vi "ziExample-Module-SWtrigger.vi"() -> ()   [LabVIEW 2009]
doc: "Control a Zurich instrument device via the LabOne Labview API. \nRequirements: Zurich Instruments MFLI, HF2 or UHFLI \nThis example shows how to start a software trigger module and retrieve the Data.\n\n© Zurich Instruments AG, www.zhinst.com"
uses:
  <instrlib>/Zurich Instruments LabOne/Public/Modules/ziModSetValueBinary.vi
  <instrlib>/Zurich Instruments LabOne/Public/Configure/ziSetValueDoubleArray.vi
  <instrlib>/Zurich Instruments LabOne/Public/Modules/ziModSetValueDouble.vi
  <instrlib>/Zurich Instruments LabOne/Public/Modules/ziModGetAuxinData.vi
  <instrlib>/Zurich Instruments LabOne/Public/Modules/ziModGetCounterData.vi
  <instrlib>/Zurich Instruments LabOne/Public/Modules/ziModGetDemodData.vi
  <instrlib>/Zurich Instruments LabOne/Public/Utility/ziTicksToS_vector.vi
  <instrlib>/Zurich Instruments LabOne/Public/Utility/ziTicksToS_single.vi
  <instrlib>/Zurich Instruments LabOne/Public/Modules/ziModGetImpedanceData.vi
  <instrlib>/Zurich Instruments LabOne/Zurich Instruments LabOne.lvlib
panel:
  out "Slide":dbl(slide) scale=0.0..1.0
  in  "subscribe":string="demods/0/sample"
  out "Grid DEMOD X":dbl[][](graph)
  out "Error Out":errorcluster
  in  "stop":bool
  in  "run":bool caption="Run"
  in  "TriggerModulSetup":T1={"holdoff/time"=0.2, "holdoff/count"=0.0, "delay"=-0.00125, "duration"=0.01, "pulse/min"=0.0, "pulse/max"=0.0, "type"=1, "edge"=1, "count"=5.0, "bits"=1.0, "bitmask"=1.0, "triggernode"="demods/0/sample.R", "bandwidth"=0.0, "hysteresis"=0.003, "level"=0.03, "grid/mode"=0.0, "grid/operation"=0.0, "grid/cols"=100, "grid/rows"=100, "grid/direction"=0.0, "grid/repetitions"=1.0} {"grid/direction" items=["Forward", "Reverse", "Bi-directional"]; "grid/operation" items=["Replace", "Average"]; "grid/mode" items=["OFF", "Nearest", "Linear"]; "level" format="%#_6p"; "hysteresis" format="%#_6p"; "bandwidth" format="%#_6p"; "edge" items=["positive"=1, "negative"=2, "both"=3]; "type" items=["edge"=1, "digital"=2, "pulse"=3, "tracking edge"=4, "HW Trigger"=6, "tracking pulse"=7]}
  out "Demod X":T2(graph)
  in  "Address":string="DEV"
  out "Selected Device":string
  # "ziExample-SweepModul.vi\nRequirements: \n- HF2LI, UHFLI or MFLI \n- MD Option\nsee block diagram for VI description"
  # "Tested Instruments:\n- HF2LI\n- UHFLI\n- MFLI"
  # "Trigger Settings"
  # "edge/pulse/tracking edge/tracking pulse"
  # "only for tracking mode"
  # "digital"
  # "Horizontal"
  # "only for pulse/tracking pulse"
  # "only for pulse/tracking pulse"
  # "Grid Mode"
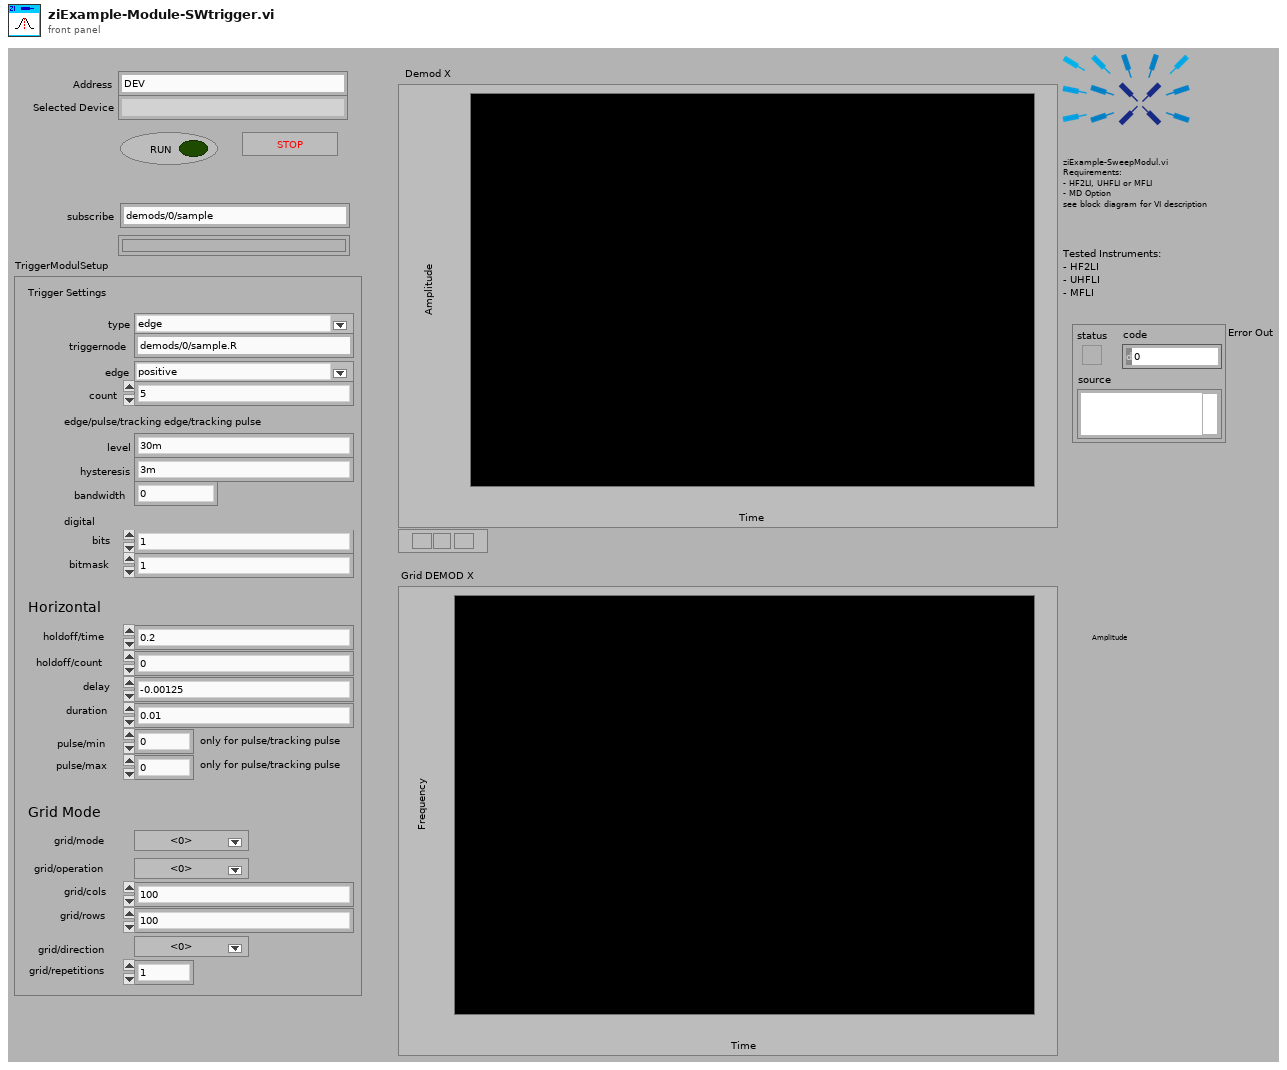
[diagram p1: front panel]
types:
  T1 = cluster{"holdoff/time":dbl, "holdoff/count":dbl, "delay":dbl, "duration":dbl, "pulse/min":dbl, "pulse/max":dbl, "type":u16, "edge":u16, "count":dbl, "bits":dbl, "bitmask":dbl, "triggernode":string, "bandwidth":dbl, "hysteresis":dbl, "level":dbl, "grid/mode":dbl, "grid/operation":dbl, "grid/cols":u32, "grid/rows":u32, "grid/direction":dbl, "grid/repetitions":dbl}
  T2 = cluster{"Timestamp(s)":dbl[], "X (Vrms)":dbl[]}[]
  T3 = typedef "Zurich Instruments LabOne.lvlib/ziTypeHandle.ctl" = cluster{"handleValid":bool, "Conn":u64, "Path Prefix":string, "Handle":u64, "Connected":bool, "Clockbase(s)":dbl}
  T4 = typedef "Zurich Instruments LabOne.lvlib/ziTypeModHandle.ctl" = cluster{"handleValid":bool, "Conn":u64, "ModHandle":u64, "moduleID":string, "Path Prefix":string}
  T5 = typedef "Zurich Instruments LabOne.lvlib/ziTypeModResults.ctl" = cluster{"PathArray":string[], "ValueType":T6, "NoOfResults":u64, "HeaderType":enum16{"HEADER_TYPE_NONE", "HEADER_TYPE_SWTRIGGER", "HEADER_TYPE_SWEEPER"}, "ziSWTriggerHeader":T7[], "ziSweeperHeader":T8[]}
  T6 = typedef "Zurich Instruments LabOne.lvlib/ziTypePollType.ctl" = enum16{"NONE", "DOUBLE_DATA", "INTEGER_DATA", "DEMOD_SAMPLE", "SCOPE_WAVE_HF2", "AUXIN_SAMPLE", "DIO_SAMPLE", "BYTE_ARRAY", "PWA_WAVE", "9", "10", "11", "12", "13", "14", "15", "TREE_CHANGE_DEPRI", "17", "ERROR", "19", "20", "21", "22", "23", "24", "25", "26", "27", "28", "29", "30", "31", "DOUBLE_DATA_TS", "INTEGER_DATA_TS", "34", "SCOPE_WAVE", "36", "37", "BYTE_ARRAY_TS", "39", "40", "41", "42", "43", "44", "45", "CNT_DATA", "47", "TREE_CHANGE", "49", "50", "51", "52", "53", "54", "55", "56", "57", "58", "59", "60", "61", "62", "63", "SWEEPER_DATA", "SPECTRUM_DATA", "ADVISOR_DATA", "67", "IMP_DATA"}
  T7 = typedef "Zurich Instruments LabOne.lvlib/ziTypeModSWTriggerHeader.ctl" = cluster{"HeaderType":enum8{"HEADER_TYPE_NONE", "HEADER_TYPE_SWTRIGGER", "HEADER_TYPE_SWEEPER"}, "triggerStart":u64, "triggerNumber":u64, "cols":u32, "rows":u32}
  T8 = typedef "Zurich Instruments LabOne.lvlib/ziTypeModSweeperHeader.ctl" = cluster{"HeaderType":enum8{"HEADER_TYPE_NONE", "HEADER_TYPE_SWTRIGGER", "HEADER_TYPE_SWEEPER"}, "sampleFormat":u8}
  T9 = typedef "ziTypeDemodSampleExGrid.ctl" = cluster{"Timestamps (ticks)":u64[][], "X (Vrms)":dbl[][], "Y (Vrms)":dbl[][], "Osc Phase (rad)":dbl[][], "Freq (Hz)":dbl[][], "DIO":u32[][], "Aux In 0 (V)":dbl[][], "Aux In 1 (V)":dbl[][], "Trigger":u32[][]}
  T10 = typedef "ziTypeDemodSampleEx.ctl" = cluster{"Timestamps (ticks)":u64[], "X (Vrms)":dbl[], "Y (Vrms)":dbl[], "Osc Phase (rad)":dbl[], "Freq (Hz)":dbl[], "DIO":u32[], "Aux In 0 (V)":dbl[], "Aux In 1 (V)":dbl[], "Trigger":u32[]}
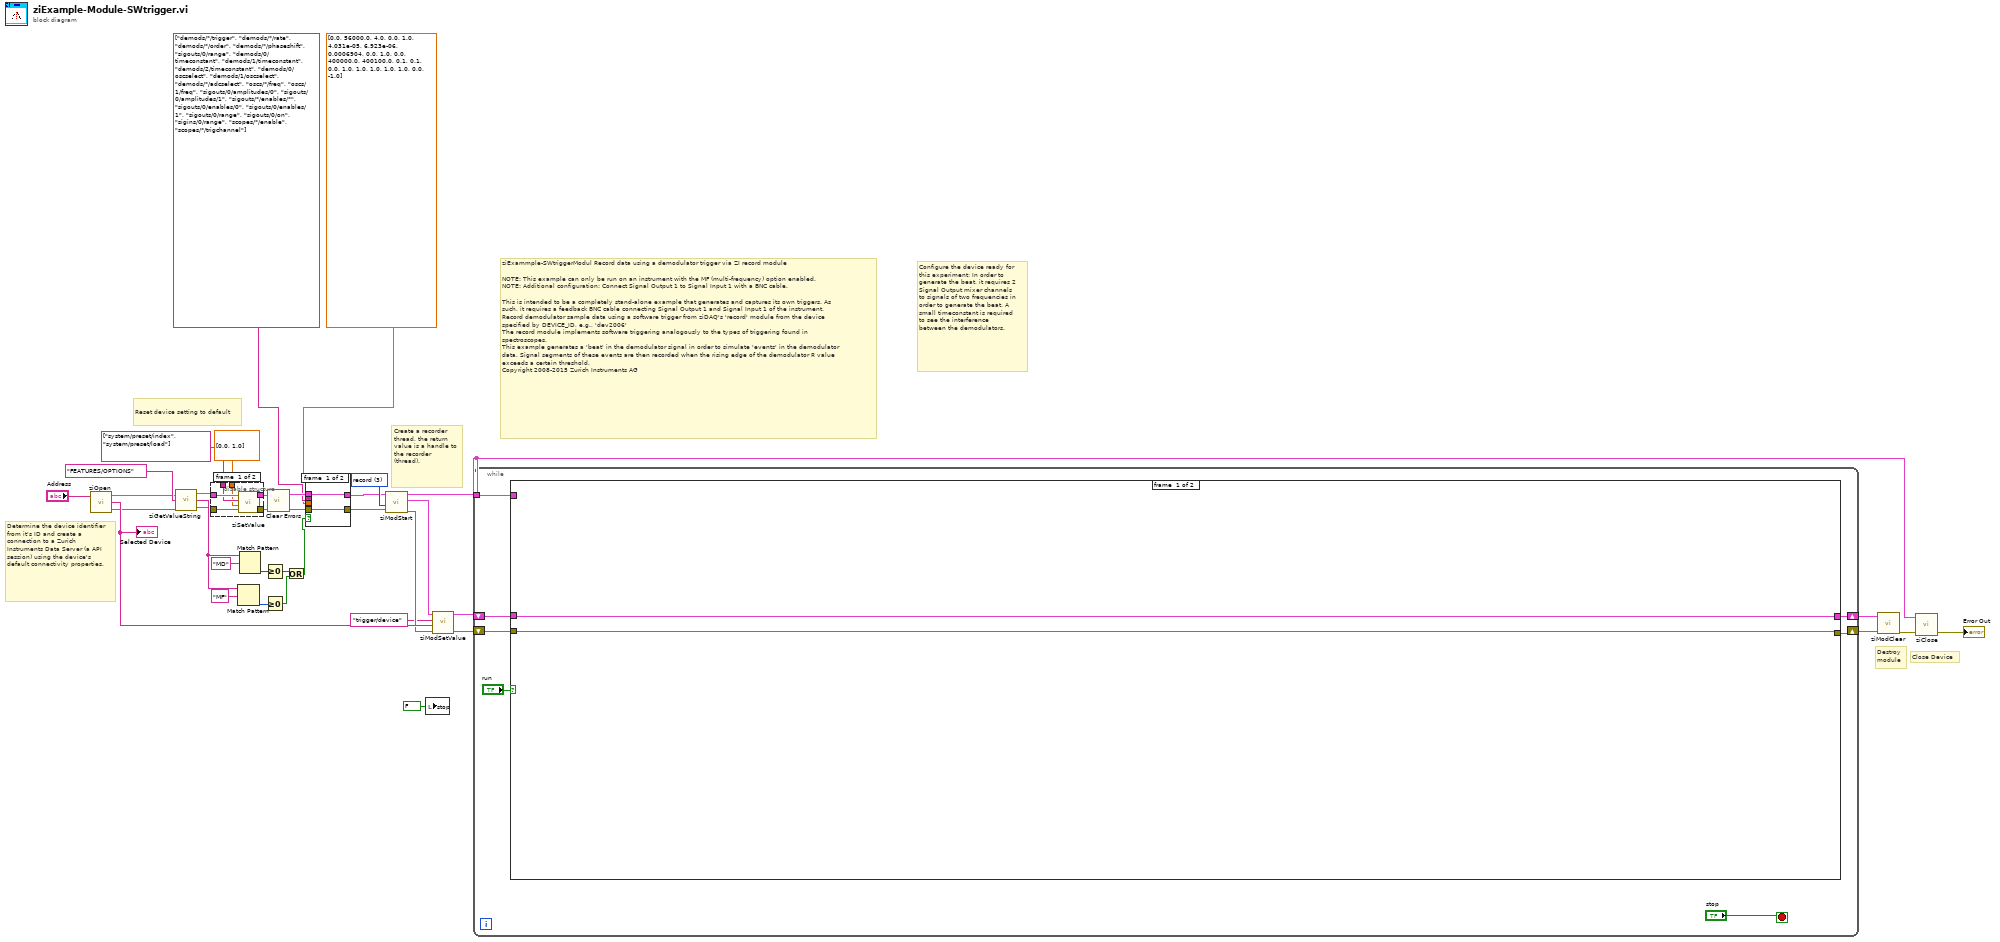
[diagram p0: block diagram]
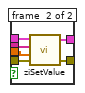
[diagram p2: hidden frame]
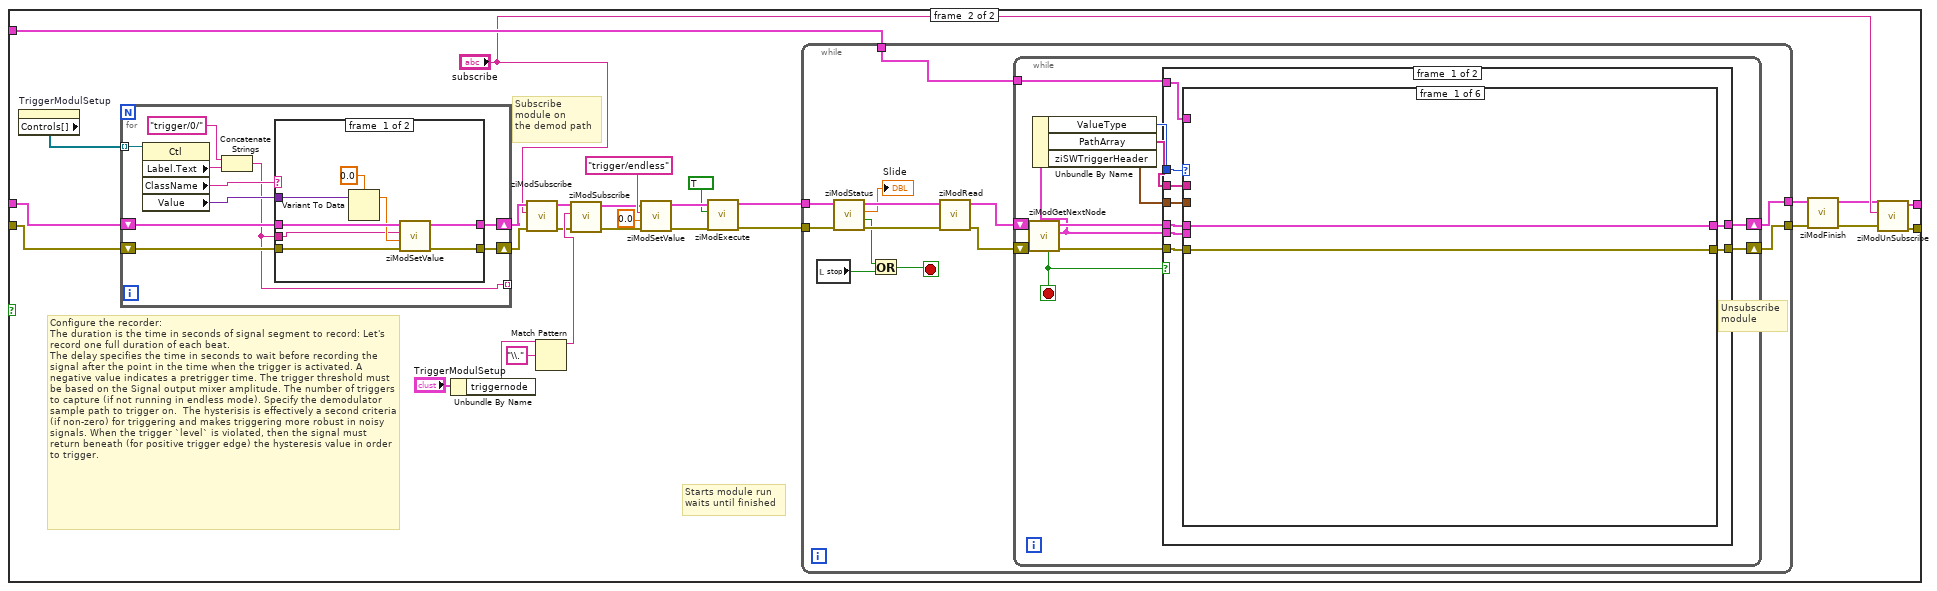
[diagram p4: hidden frame]
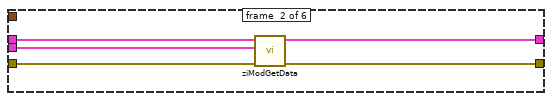
[diagram p5: hidden frame]
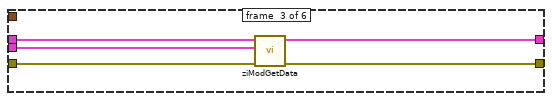
[diagram p6: hidden frame]
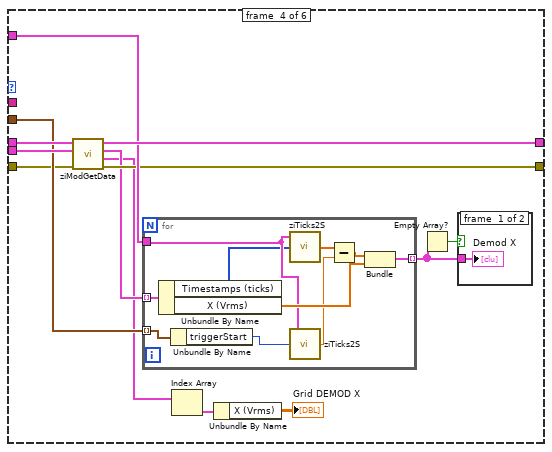
[diagram p7: hidden frame]
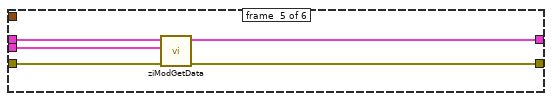
[diagram p9: hidden frame]
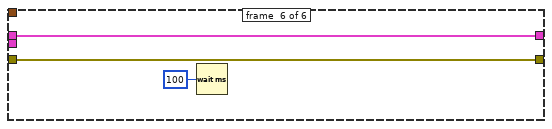
[diagram p10: hidden frame]
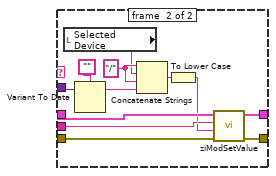
[diagram p12: hidden frame]
diagram:
  w34 = u16 3 items=["sweep", "zoomFFT", "deviceSettings", "record", "pllAdvisor", "pidAdvisor"] ("moduleID")
  # "ziExammple-SWtriggerModul Record data using a demodulator trigger via ZI record module\n\nNOTE: This example can only be run on an instrument with the MF (multi-frequency) option enabled. \nNOTE: Additional configuration: Connect Signal Output 1 to Signal Input 1 with a BNC cable.\n\nThis is intended to be a completely stand-alone example that generates and captures its own triggers. As such, it requires a feedback BNC cable connecting Signal Output 1 and Signal Input 1 of the instrument.\nRecord demodulator sample data using a software trigger from ziDAQ's 'record' module from the device specified by DEVICE_ID, e.g., 'dev2006' \nThe record module implements software triggering analogously to the types of triggering found in spectroscopes.\nThis example generates a 'beat' in the demodulator signal in order to simulate 'events' in the demodulator data. Signal segments of these events are then recorded when the rising edge of the demodulator R value exceeds a certain threshold.\nCopyright 2008-2015 Zurich Instruments AG"
  # "Configure the device ready for this experiment: In order to generate the beat, it requires 2 Signal Output mixer channels to signals of two frequencies in order to generate the beat. A small timeconstant is required to see the interference between the demodulators."
  # "Reset device setting to default"
  # "Destroy\nmodule"
  # "Create a recorder thread, the return value is a handle to the recorder (thread)."
  # "Close Device"
  # "Determine the device identifier from it's ID and create a connection to a Zurich Instruments Data Server (a API session) using the device's default connectivity properties."
  n1 = call <instrlib>:"ziOpen.vi"("Address"="Address") -> ("Error Out"=w5:errorcluster, "Selected Device"=w35:string, "HandleOut"=w4:T3)  [unwired: 1 in, 2 out]
  "Selected Device" <- w35
  n2 = call <instrlib>:"ziGetValueString.vi"("error in"=w5, "Path"="FEATURES/OPTIONS", "Handle In"=w4) -> ("error out"=w2:errorcluster, "Value"=w10:string, "Handle Out"=w3:T3)
  n3 = disable-structure shown="Enabled" {
    disable-tunnel: w3 -> [w42 w44]
    disable-tunnel: [w41 w44] -> w27
    disable-tunnel: [w40 w43] -> w26
    disable-tunnel: w2 -> [w39 w43]
    disable-tunnel: string[] ["system/preset/index", "system/preset/load"] -> [w38 _]
    disable-tunnel: dbl[] [0.0, 1.0] -> [w37 _]
    frame #0 {
      n4 = call-poly <instrlib>:"ziSetValue.vi"("Error In"=w39, "Values"=w37, "Paths"=w38, "Handle In"=w42) -> ("Error Out"=w40:errorcluster, "Handle Out"=w41:T3)  [unwired: 1 in]
    }
    frame #1 {
    }
  }
  n5 = Match Pattern(string=w10, regular expression="MF") -> (offset past match=w8:i32)  [unwired: 1 in, 3 out]
  n6 = Match Pattern(string=w10, regular expression="MD") -> (offset past match=w11:i32)  [unwired: 1 in, 3 out]
  n7 = Greater Or Equal To 0?(x=w11) -> (x >= 0?=w7:bool)
  n8 = Greater Or Equal To 0?(x=w8) -> (x >= 0?=w6:bool)
  n9 = call <vilib>:"Clear Errors.vi"("error in (no error)"=w26) -> ("error out"=w16:errorcluster)  [unwired: 6 in]
  n10 = Or(x=w7, y=w6) -> (x .or. y?=w1:bool)
  n11 = case shown="True" w1 {
    tunnel: [w46 w52] -> w30
    tunnel: [w45 w51] -> w29
    tunnel: w27 -> [w46 w50]
    tunnel: string[] ["demods/*/trigger", "demods/*/rate", "demods/*/order", "demods/*/phaseshift", "sigouts/0/range", "demods/0/timeconstant", "demods/1/timeconstant", "demods/2/timeconstant", "demods/0/oscselect", "demods/1/oscselect", "demods/*/adcselect", "oscs/*/freq", "oscs/1/freq", "sigouts/0/amplitudes/0", "sigouts/0/amplitudes/1", "sigouts/*/enables/*", "sigouts/0/enables/0", "sigouts/0/enables/1", "sigouts/0/range", "sigouts/0/on", "sigins/0/range", "scopes/*/enable", "scopes/*/trigchannel"] -> [_ w49]
    tunnel: dbl[] [0.0, 56000.0, 4.0, 0.0, 1.0, 4.031e-05, 6.923e-06, 0.0006904, 0.0, 1.0, 0.0, 400000.0, 400100.0, 0.1, 0.1, 0.0, 1.0, 1.0, 1.0, 1.0, 1.0, 0.0, -1.0] -> [_ w48]
    tunnel: w16 -> [w45 w47]
    frame #0 {
    }
    frame #1 {
      n12 = call-poly <instrlib>:"ziSetValue.vi"("Error In"=w47, "Values"=w48, "Paths"=w49, "Handle In"=w50) -> ("Error Out"=w51:errorcluster, "Handle Out"=w52:T3)  [unwired: 1 in]
    }
  }
  n13 = call <instrlib>:"ziModStart.vi"("Error In"=w29, "module Id"=w34, "Handle In"=w30) -> ("Error Out"=w32:errorcluster, "ModHandle Out"=w33:T4, "Handle Out"=w24:T3)  [unwired: 6 in]
  n14 = local write "stop"(FALSE ("stop")) -> ()
  n15 = call-poly <instrlib>:"ziModSetValue.vi"("Error In"=w32, "Data"=w35, "Path"="trigger/device", "ModHandle In"=w33) -> ("Error Out"=w25:errorcluster, "ModHandle Out"=w15:T4)  [unwired: 6 in]
  n16 = while {
    tunnel: w24 -> [w59]
    shift-right: [w54] -> w22
    shift-left: w15 -> [w58]
    shift-right: [w53] -> w23
    shift-left: w25 -> [w57]
    stop <- "stop" stop-if-true
    n17 = case shown="True" "run" {
      tunnel: [w60 w78] -> w54
      tunnel: [w61 w79] -> w53
      tunnel: w59 -> [_ w87]
      tunnel: w58 -> [w60 w83]
      tunnel: w57 -> [w61 w82]
      frame #0 {
      }
      frame #1 {
        # "Starts module run\nwaits until finished"
        # "Configure the recorder:\nThe duration is the time in seconds of signal segment to record: Let's record one full duration of each beat.\nThe delay specifies the time in seconds to wait before recording the signal after the point in the time when the trigger is activated. A negative value indicates a pretrigger time. The trigger threshold must be based on the Signal output mixer amplitude. The number of triggers to capture (if not running in endless mode). Specify the demodulator sample path to trigger on.  The hysterisis is effectively a second criteria (if non-zero) for triggering and makes triggering more robust in noisy signals. When the trigger `level` is violated, then the signal must return beneath (for positive trigger edge) the hysteresis value in order to trigger."
        # "Subscribe\nmodule on\nthe demod path"
        n18 = property on="TriggerModulSetup" class="Clust (strict)"() -> ("Controls[]"=w86:refnum<vi>[])  [unwired: 2 in, 2 out]
        n19 = for {
          tunnel: w86 -> [w179] mode=indexing
          shift-right: [w173] -> w84
          shift-left: w82 -> [w171]
          shift-right: [w174] -> w85
          shift-left: w83 -> [w172]
          tunnel: [w170] -> _ mode=indexing
          n20 = property class="Ctl"(reference=w179) -> ("Label.Text"=w177:string, "ClassName"=w176:string, "Value"=w175:variant)  [unwired: 1 in, 2 out]
          n21 = Concatenate Strings("trigger/0/" ("string"), w177) -> (w170:string)
          n22 = case shown="\"String\"" w176 {
            tunnel: w170 -> [w180 w193]
            tunnel: w175 -> [w187 w198]
            tunnel: [w184 w197] -> w174
            tunnel: [w183 w196] -> w173
            tunnel: w172 -> [w185 w195]
            tunnel: w171 -> [w182 w194]
            frame #0 {
              n23 = Variant To Data(Variant=w187, type=0.0) -> (data=w181:dbl)  [unwired: 1 in, 1 out]
              n24 = call-poly <instrlib>:"ziModSetValue.vi"("Error In"=w182, "Value"=w181, "Path"=w180, "ModHandle In"=w185) -> ("Error Out"=w183:errorcluster, "ModHandle Out"=w184:T4)  [unwired: 6 in]
            }
            frame #1 {
              w192 = "/"
              n25 = local read "Selected Device"() -> (w191:string)
              n26 = Variant To Data(Variant=w198, type="") -> (data=w190:string)  [unwired: 1 in, 1 out]
              n27 = Concatenate Strings(w192, w191, w192, w190) -> (w189:string)
              n28 = To Lower Case(string=w189) -> (all lower case string=w188:string)
              n29 = call-poly <instrlib>:"ziModSetValue.vi"("Error In"=w194, "Data"=w188, "Path"=w193, "ModHandle In"=w195) -> ("Error Out"=w196:errorcluster, "ModHandle Out"=w197:T4)  [unwired: 6 in]
            }
          }
        }
        n30 = Unbundle By Name("TriggerModulSetup") -> ("triggernode"=w72:string)
        n31 = call <instrlib>:"ziModSubscribe.vi"("Error In"=w84, "Path"="subscribe", "ModHandle In"=w85) -> ("Error Out"=w68:errorcluster, "ModHandle Out"=w69:T4)  [unwired: 6 in]
        n32 = Match Pattern(string=w72, regular expression="\\.") -> (before substring=w70:string)  [unwired: 1 in, 3 out]
        n33 = call <instrlib>:"ziModSubscribe.vi"("Error In"=w68, "Path"=w70, "ModHandle In"=w69) -> ("Error Out"=w66:errorcluster, "ModHandle Out"=w67:T4)  [unwired: 6 in]
        n34 = call-poly <instrlib>:"ziModSetValue.vi"("Error In"=w66, "Value"=0.0, "Path"="trigger/endless", "ModHandle In"=w67) -> ("Error Out"=w80:errorcluster, "ModHandle Out"=w81:T4)  [unwired: 6 in]
        n35 = call <instrlib>:"ziModExecute.vi"("Error In"=w80, "Modal (F)"=TRUE, "ziModHandle In"=w81) -> ("Error Out"=w74:errorcluster, "ziModHandle Out"=w75:T4)  [unwired: 5 in, 1 out]
        n36 = while {
          tunnel: w87 -> [w102]
          tunnel: w75 -> [w97]
          tunnel: w74 -> [w96]
          tunnel: [w95] -> w64
          tunnel: [w94] -> w63
          stop <- w90 stop-if-true
          # "Unsubscribe\nmodule"
          n37 = local read "stop"() -> (w92:bool)
          n38 = call <instrlib>:"ziModStatus.vi"("Error In"=w96, "ModHandle IN"=w97) -> ("Error Out"=w98:errorcluster, "Finished?"=w91:bool, "Progress (unity)"=→"Slide":dbl, "ModHandle Out"=w99:T4)  [unwired: 5 in]
          n39 = Or(x=w91, y=w92) -> (x .or. y?=w90:bool)
          n40 = call <instrlib>:"ziModRead.vi"("error in"=w98, "ziModHandle In"=w99) -> ("error out"=w101:errorcluster, "ziModHandle Out"=w100:T4)  [unwired: 8 in]
          n41 = while {
            shift-right: [w109] -> w94
            shift-left: w100 -> [w113]
            shift-right: [w110] -> w95
            shift-left: w101 -> [w114]
            tunnel: w102 -> [w108]
            stop <- w106 stop-if-true
            # "Retrieve results"
            n42 = call <instrlib>:"ziModGetNextNode.vi"("Error In"=w114, "ModHandle In"=w113) -> ("Error Out"=w111:errorcluster, "ModResults"=w104:T5, "ModHandle Out"=w112:T4, "NoData"=w106:bool)  [unwired: 6 in]
            n43 = Unbundle By Name(w104) -> ("ValueType"=w105:T6, "PathArray"=w107:string[], "ziSWTriggerHeader"=w103:T7[])
            n44 = case shown="False" w106 {
              tunnel: w104 -> [w123 _]
              tunnel: w112 -> [w122 w169]
              tunnel: w111 -> [w121 w168]
              tunnel: [w120 w168] -> w110
              tunnel: [w119 w169] -> w109
              tunnel: w105 -> [w118 _]
              tunnel: w108 -> [w117 _]
              tunnel: w107 -> [w116 _]
              tunnel: w103 -> [w115 _]
              frame #0 {
                n45 = case shown="\"DEMOD_SAMPLE\"" w118 {
                  tunnel: w122 -> [w125 w130 w135 w145 w162 w167]
                  tunnel: w123 -> [_ w128 w133 w146 w163 _]
                  tunnel: w121 -> [w124 w129 w134 w141 w160 w166]
                  tunnel: [w124 w126 w131 w144 w161 w166] -> w120
                  tunnel: [w125 w127 w132 w148 w164 w167] -> w119
                  tunnel: w117 -> [_ _ _ w147 _ _]
                  tunnel: w116 -> [_ _ _ _ _ _]
                  tunnel: w115 -> [_ _ _ w142 _ _]
                  frame #0 {
                  }
                  frame #1 {
                    n46 = call-poly <instrlib>:"ziModGetData.vi"("Error In"=w129, "ModResults"=w128, "ModHandle In"=w130) -> ("Error Out"=w126:errorcluster, "ModHandle Out"=w127:T4)  [unwired: 5 in, 2 out]
                  }
                  frame #2 {
                    n47 = call-poly <instrlib>:"ziModGetData.vi"("Error In"=w134, "ModResults"=w133, "ModHandle In"=w135) -> ("Error Out"=w131:errorcluster, "ModHandle Out"=w132:T4)  [unwired: 6 in, 1 out]
                  }
                  frame #3 {
                    n48 = call-poly <instrlib>:"ziModGetData.vi"("Error In"=w141, "ModResults"=w146, "ModHandle In"=w145) -> ("Error Out"=w144:errorcluster, "ModDemodDataGrid"=w140:T9[], "ModDemodData"=w143:T10[], "ModHandle Out"=w148:T4)  [unwired: 5 in]
                    n49 = for {
                      tunnel: w143 -> [w159] mode=indexing
                      tunnel: [w157] -> w137 mode=indexing
                      tunnel: w147 -> [w154]
                      tunnel: w142 -> [w156] mode=indexing
                      n50 = Unbundle By Name(w159) -> ("Timestamps (ticks)"=w152:u64[], "X (Vrms)"=w158:dbl[])
                      n51 = Unbundle By Name(w156) -> ("triggerStart"=w155:u64)
                      n52 = call-poly <instrlib>:"ziTicks2S.vi"("Timestamp (ticks)"=w152, "Handle In"=w154) -> ("Timestamp(s)"=w151:dbl[])  [unwired: 1 in, 2 out]
                      n53 = call-poly <instrlib>:"ziTicks2S.vi"("Timestamp(ticks)"=w155, "Handle In"=w154) -> ("Timestamp(s)"=w153:dbl)  [unwired: 1 in, 2 out]
                      n54 = Subtract(x=w151, y=w153) -> (x-y=w150:dbl[])
                      n55 = Bundle(w150, "X (Vrms)"=w158) -> (w157:cluster{dbl[], "X (Vrms)":dbl[]})  [unwired: 1 in]
                    }
                    n56 = Index Array(array=w140) -> (element=w139:T9)  [unwired: 1 in]
                    n57 = Unbundle By Name(w139) -> ("X (Vrms)"=→"Grid DEMOD X":dbl[][])
                    n58 = Empty Array?(array=w137) -> (empty?=w136:bool)
                    n59 = case shown="False" w136 {
                      tunnel: w137 -> [w149 _]
                      frame #0 {
                        "Demod X" <- w149
                      }
                      frame #1 {
                      }
                    }
                  }
                  frame #4 {
                    n60 = call-poly <instrlib>:"ziModGetData.vi"("Error In"=w160, "ModResults"=w163, "ModHandle In"=w162) -> ("Error Out"=w161:errorcluster, "ModHandle Out"=w164:T4)  [unwired: 5 in, 2 out]
                  }
                  frame #5 {
                    n61 = Wait (ms)(milliseconds to wait=u32 100) -> ()  [unwired: 1 out]
                  }
                }
              }
              frame #1 {
              }
            }
          }
        }
        n62 = call <instrlib>:"ziModFinish.vi"("Error In"=w64, "ziModHandle In"=w63) -> ("Error Out"=w65:errorcluster, "ziModHandle Out"=w62:T4)  [unwired: 7 in]
        n63 = call <instrlib>:"ziModUnSubscribe.vi"("Error In"=w65, "Path (\"/\")"="subscribe", "ModHandle In"=w62) -> ("Error Out"=w79:errorcluster, "ModHandle Out"=w78:T4)  [unwired: 7 in]
      }
    }
  }
  n64 = call <instrlib>:"ziModClear.vi"("Error In"=w23, "ziModHandle In"=w22) -> ("Error Out"=w36:errorcluster)  [unwired: 7 in, 1 out]
  n65 = call <instrlib>:"ziClose.vi"("Error In"=w36, "Handle In"=w24) -> ("Error Out"=→"Error Out":errorcluster)  [unwired: 2 in, 1 out]
